vi "OSC Availables.vi"(8 "error in":errorcluster, 10 "OSC Type":string[](array[string]), 11 "Module ID":i32=-1) -> (0 "error out":errorcluster)   [LabVIEW 2020, in "Oscilloscope.lvlib"]
doc: "_____\nCreated using DQMH Event Scripter 6.0.0.122."
uses:
  Oscilloscope.lvlib
  OSC Availables Argument--cluster.ctl
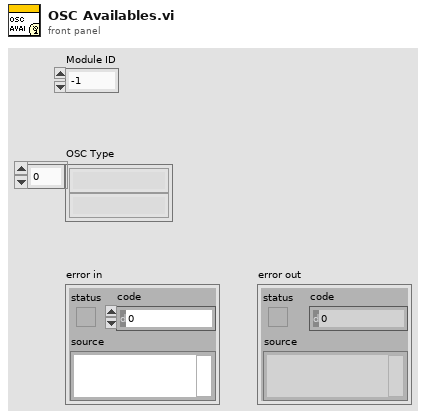
[diagram p1: front panel]
types:
  T1 = typedef "Oscilloscope.lvlib/OSC Availables Argument--cluster.ctl" = cluster{"Module ID":i32, "OSC Type":string[]}
  T2 = typedef "Oscilloscope.lvlib/Broadcast Events--cluster.ctl" = cluster{"Module Did Init":refnum<user-event>, "Status Updated":refnum<user-event>, "Error Reported":refnum<user-event>, "Module Did Stop":refnum<user-event>, "Update Module Execution Status":refnum<user-event>, "OSC Availables":refnum<user-event>}
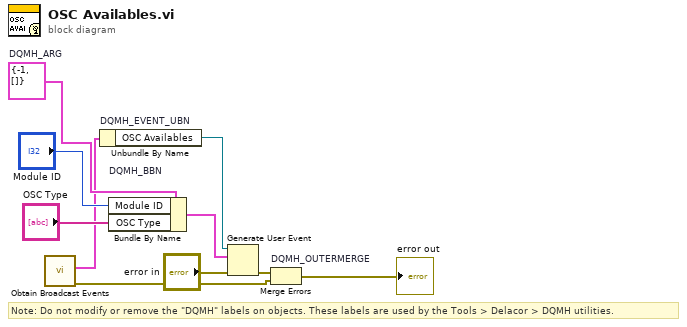
[diagram p0: block diagram]
diagram:
  w5 = T1 {"Module ID"=-1, "OSC Type"=[]}  # DQMH_ARG
  # "Note: Do not modify or remove the \"DQMH\" labels on objects. These labels are used by the Tools > Delacor > DQMH utilities."
  n1 = call "Obtain Broadcast Events.vi"() -> ("error out"=w2:errorcluster, "Oscilloscope Broadcast Events"=w1:T2)  [unwired: 10 in]
  n2 = Unbundle By Name "DQMH_EVENT_UBN"(w1) -> ("OSC Availables"=w7:refnum<user-event>)
  n3 = Bundle By Name "DQMH_BBN"(cluster=w5, "Module ID"="Module ID", "OSC Type"="OSC Type") -> (w8:T1)
  n4 = Generate User Event(user event=w7, event data cluster=w8, error in="error in") -> (error out=w6:errorcluster)  [unwired: 1 in, 1 out]
  n5 = Merge Errors "DQMH_OUTERMERGE"(w6, w2) -> (→"error out":errorcluster)
